vi "Update Routed State.vi"(8 "error in (no error)":errorcluster, 10 "Set":bool, 11 "MLTFNC in":refnum<class "MLTFNC.lvclass">) -> (0 "error out":errorcluster, 3 "MLTFNC out":refnum<class "MLTFNC.lvclass">)   [LabVIEW 2019, in "MLTFNC.lvlib" / "MLTFNC.lvclass"]
uses:
  Library/MLTFNC.lvclass
  Library/MLTFNC.lvclass/MLTFNC.ctl
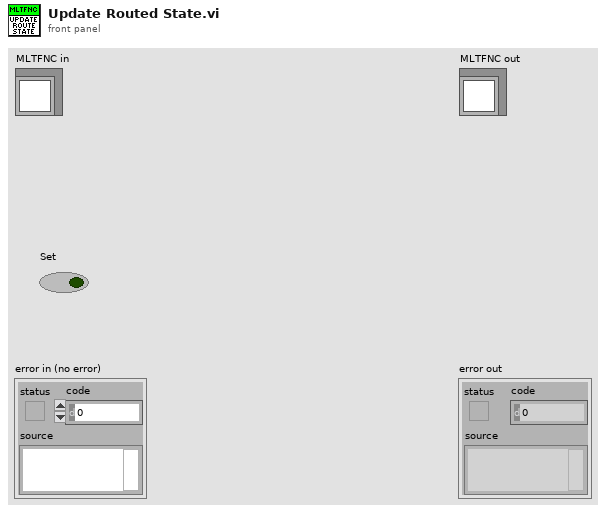
[diagram p1: front panel]
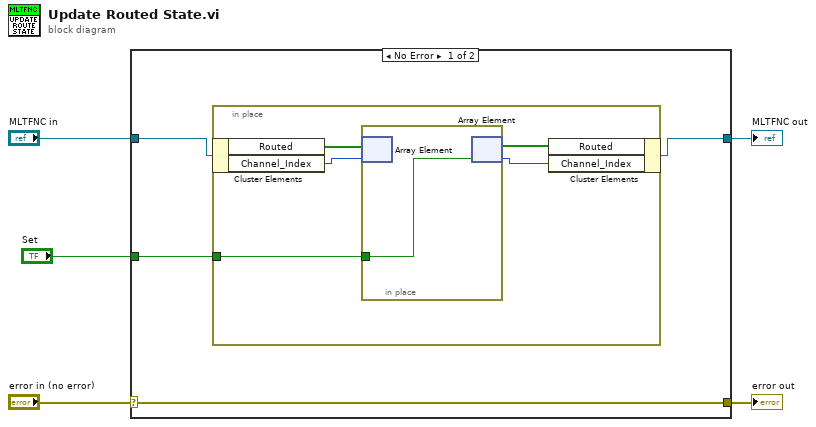
[diagram p0: block diagram]
diagram:
  n1 = case shown="No Error" "error in (no error)" {
    selector: "error in (no error)" -> [w9 w17]
    tunnel: [w9 w17] -> w4
    tunnel: [w7 w16] -> w2
    tunnel: "MLTFNC in" -> [w8 w16]
    tunnel: "Set" -> [w6 _]
    frame No Error {
      n2 = in-place {
        in-place-border: w6 -> [w10]
        n3 = in-place-cluster #1(w8) -> ("Routed"=w14:bool[], "Channel_Index"=w13:i32)
        n4 = in-place {
          in-place-border: w10 -> [w15]
          n5 = in-place-array #2(w14, w13) -> ()  [unwired: 1 out]
          n6 = in-place-array #2(w15) -> (w12:bool[], w11:i32)
        }
        n7 = in-place-cluster #1("Routed"=w12, "Channel_Index"=w11) -> (w7:refnum<class "MLTFNC.lvclass">)
      }
    }
    frame Error {
    }
  }
  "error out" <- w4
  "MLTFNC out" <- w2
